vi "ScanAction.vi"(8 "error in (no error)":errorcluster caption="entrée d'erreur (pas d'erreur)", 9 "IndicePoint":i32, 11 "Tools In":refnum<class "LeafMagnetometer.lvclass"> caption="DNL_LabVIEW Object in") -> (0 "error out":errorcluster caption="sortie d'erreur", 2 "ScanParOut":dbl, 3 "Tools Out":refnum<class "LeafMagnetometer.lvclass"> caption="DNL_LabVIEW Object out")   [LabVIEW 2010, in "LeafMagnetometer.lvclass"]
uses:
  LeafMagnetometer.lvclass
  LeafMagnetometer.lvclass/LeafMagnetometer.ctl
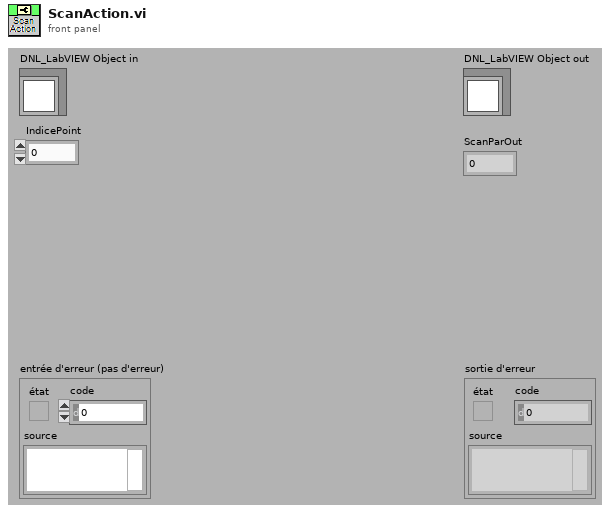
[diagram p1: front panel]
types:
  T1 = typedef "LeafMagnetometer.lvclass/LeafMagnetometer_Func.ctl" = enum16{"DefaultFunc (Arb)"}
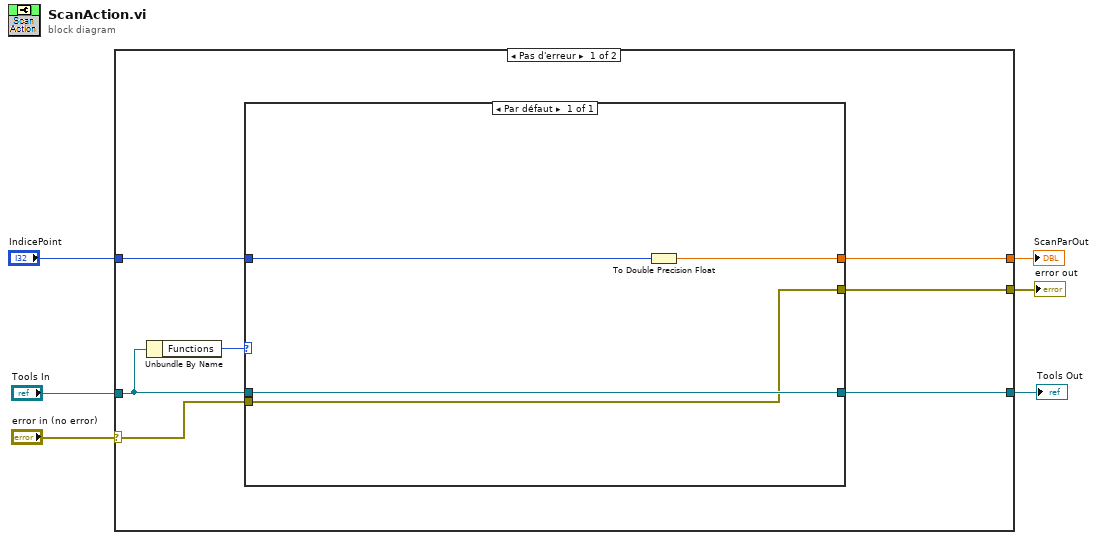
[diagram p0: block diagram]
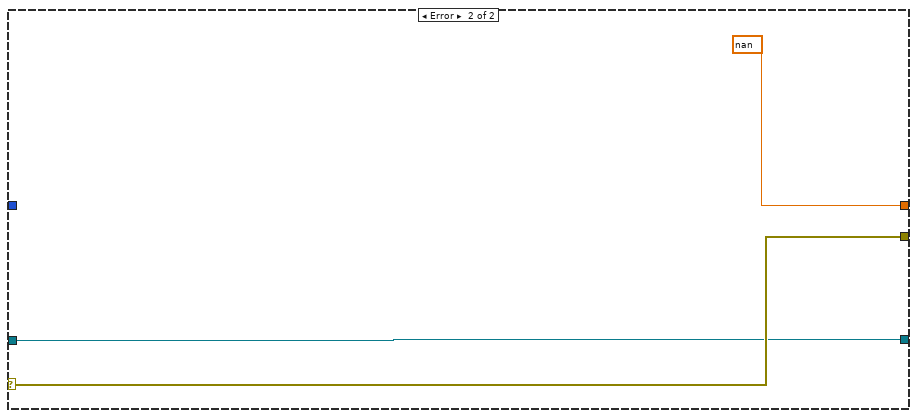
[diagram p2: hidden frame]
diagram:
  n1 = case shown="Pas d'erreur" "error in (no error)" {
    selector: "error in (no error)" -> [w10 w19]
    tunnel: "Tools In" -> [w11 w18]
    tunnel: [w9 nan ("Lambda Out (nm)")] -> w4
    tunnel: [w8 w19] -> w3
    tunnel: [w7 w18] -> w2
    tunnel: "IndicePoint" -> [w12 _]
    frame No Error {
      n2 = Unbundle By Name(w11) -> ("Functions"=w13:T1)
      n3 = case shown="Par défaut" w13 {
        tunnel: [w16] -> w9
        tunnel: w12 -> [w17]
        tunnel: [w15] -> w7
        tunnel: w11 -> [w15]
        tunnel: w10 -> [w14]
        tunnel: [w14] -> w8
        frame Par défaut {
          n4 = To Double Precision Float(number=w17) -> (double precision float=w16:dbl)
        }
      }
    }
    frame Error {
    }
  }
  "error out" <- w3
  "Tools Out" <- w2
  "ScanParOut" <- w4
